vi "parse_general_response.vi"(8 "error in (no error)":errorcluster, 10 "body":string, 11 "headers":string) -> (0 "error out":errorcluster)   [LabVIEW 2020, in "vector_qdrant.lvclass"]
uses:
  vector_qdrant.lvclass
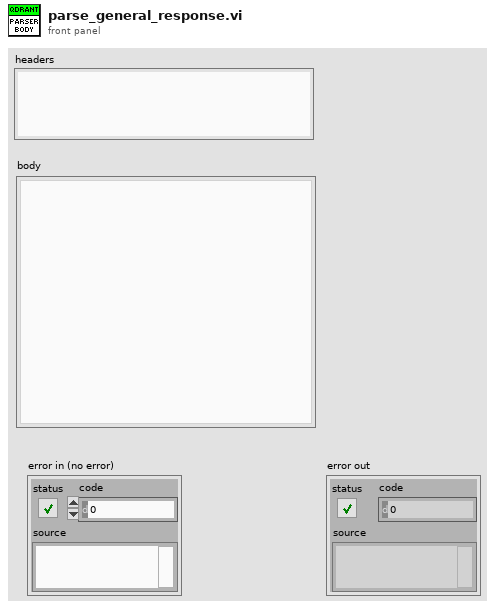
[diagram p1: front panel]
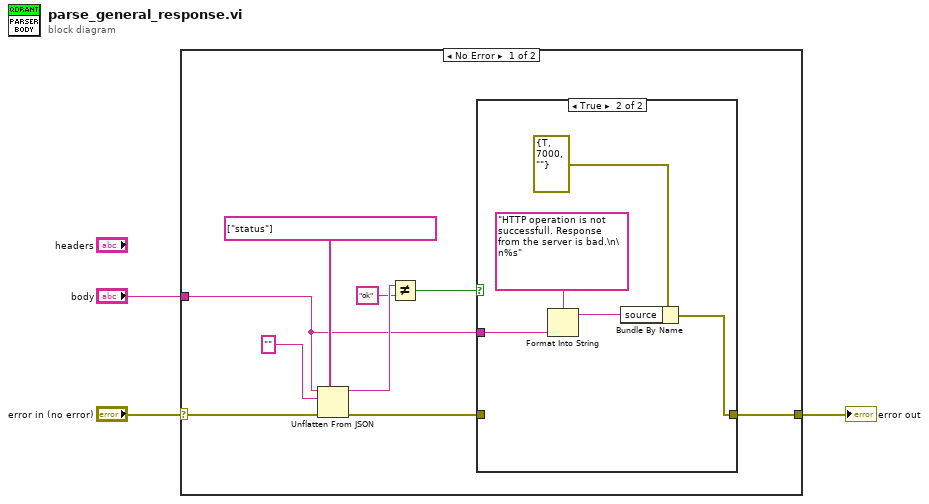
[diagram p0: block diagram]
diagram:
  n1 = case shown="No Error" "error in (no error)" {
    selector: "error in (no error)" -> [w4 w19]
    tunnel: [w6 w19] -> w3
    tunnel: "body" -> [w5 _]
    frame No Error {
      n2 = Unflatten From JSON(path=string[] ["status"], JSON string=w5, type and defaults="" ("headers"), error in (no error)=w4) -> (value=w10:string, error out=w7:errorcluster)  [unwired: 3 in]
      n3 = Not Equal?(x=w10, y="ok") -> (x != y?=w8:bool)
      n4 = case shown="True" w8 {
        tunnel: w7 -> [w13 _]
        tunnel: [w13 w17] -> w6
        tunnel: w5 -> [_ w14]
        frame False {
        }
        frame True {
          n5 = Format Into String(format string="HTTP operation is not successfull. Response from the server is bad.\n\n%s", w14) -> (resulting string=w16:string)  [unwired: 2 in, 1 out]
          n6 = Bundle By Name(cluster=errorcluster {"status"=TRUE, "code"=7000, "source"=""} ("error constant"), "source"=w16) -> (w17:errorcluster)
        }
      }
    }
    frame Error {
    }
  }
  "error out" <- w3
